vi "Do.vi"(8 "error in (no error)":errorcluster, 11 "Proto in":refnum<class "Proto.lvclass">) -> (0 "error out":errorcluster, 3 "Proto out":refnum<class "Proto.lvclass">)   [LabVIEW 2020, in "Proto.lvclass"]
uses:
  Proto.lvclass
  Proto.lvclass/Proto.ctl
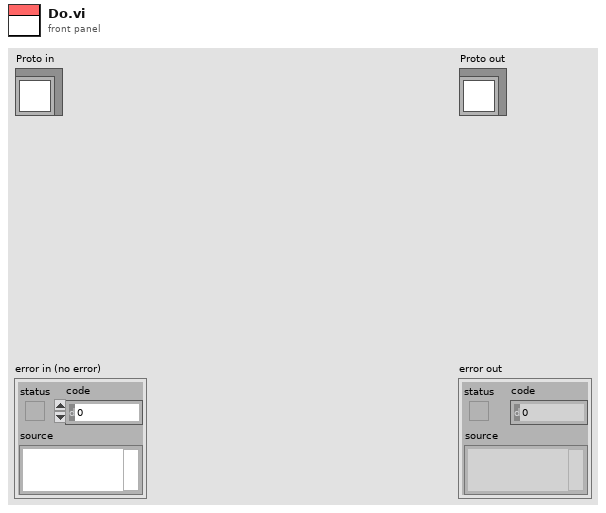
[diagram p1: front panel]
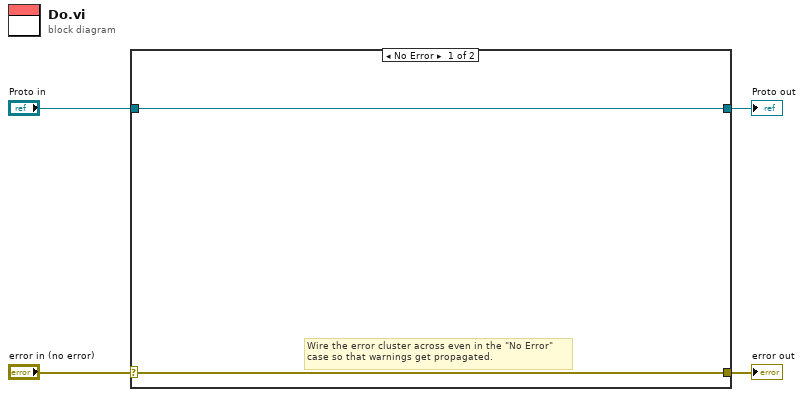
[diagram p0: block diagram]
diagram:
  n1 = case shown="No Error" "error in (no error)" {
    selector: "error in (no error)" -> [w5 w8]
    tunnel: [w5 w8] -> w3
    tunnel: [w6 w7] -> w1
    tunnel: "Proto in" -> [w6 w7]
    frame No Error {
      # "Wire the error cluster across even in the \"No Error\"\ncase so that warnings get propagated."
    }
    frame Error {
    }
  }
  "error out" <- w3
  "Proto out" <- w1
